vi "MoAgSy_Host_GPG_getPubKey.vi"(0 "Host_Reference":refnum<class "HGF_Reference.lvclass">, 5 "error in (no error)":errorcluster, 6 "timeout in ms (-1)":i32=-1) -> (14 "dup Host_Reference":refnum<class "HGF_Reference.lvclass">, 16 "public Key":string, 19 "error out":errorcluster)   [LabVIEW 2009, in "MoAgSy.lvlib" / "MoAgSy_Host.lvclass"]
doc: "<b>public</b> get Hosts publik key\n\nF.Berck@gsi.de\nGSI Darmstadt 2009"
uses:
  MoAgSy_Host.lvclass
  HGF_BaseClasses/HGF_Reference/HGF_Reference.lvclass
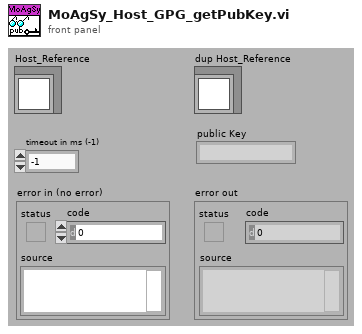
[diagram p1: front panel]
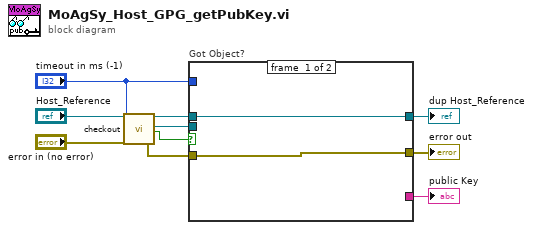
[diagram p0: block diagram]
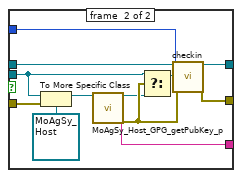
[diagram p2: hidden frame]
diagram:
  n1 = call "checkout.vi"("HGF_Reference"="Host_Reference", "timeout in ms (-1)"="timeout in ms (-1)", "error in (no error)"="error in (no error)") -> ("dup HGF_Reference"=w7:refnum<class "HGF_Reference.lvclass">, "Object"=w4:refnum<class>, "got object?"=w6:bool, "error out"=w3:errorcluster)  [unwired: 13 out]
  n2 = case "Got Object?" shown="True" w6 {
    tunnel: w3 -> [w11 w23]
    tunnel: w4 -> [_ w17]
    tunnel: w7 -> [w12 w21]
    tunnel: [w12 w20] -> w8
    tunnel: "timeout in ms (-1)" -> [_ w19]
    tunnel: [w11 w18] -> w10
    tunnel: [_ w13] -> w1
    frame #0 {
    }
    frame #1 {
      n3 = To More Specific Class(target class=refnum<class "MoAgSy_Host.lvclass"> refnum ("MoAgSy.lvlib:MoAgSy_Host.lvclass"), reference=w17, error in=w23) -> (specific class reference=w15:refnum<class "MoAgSy_Host.lvclass">)  [unwired: 1 out]
      n4 = call "MoAgSy_Host_GPG_getPubKey_p.vi"("MoAgSy_Host"=w15) -> ("dup MoAgSy_Host"=w14:refnum<class "MoAgSy_Host.lvclass">, "public Key"=w13:string, "error out"=w24:errorcluster)  [unwired: 16 in]
      n5 = Select(t=w17, s=w24, f=w14) -> (s? t:f=w16:refnum<class>)
      n6 = call "checkin.vi"("HGF_Reference"=w21, "Object"=w16, "timeout /ms (-1)"=w19, "error in (no error)"=w24) -> ("dup HGF_Reference"=w20:refnum<class "HGF_Reference.lvclass">, "error out"=w18:errorcluster)  [unwired: 14 out]
    }
  }
  "dup Host_Reference" <- w8
  "error out" <- w10
  "public Key" <- w1
